vi "INI read synchronization.vi"(11 "error in (no error)":T2) -> (4 "Sync mode":T1, 6 "Trig sync en":bool, 8 "LO sync en":bool, 15 "error out":T2)   [LabVIEW 2019, in "Shared.lvlib"]
doc: "Read mmWave LOs to export"
uses:
  Shared.lvlib
  mmWave instrument_class/Sync mode.ctl
  Low-level/TypeDefs/TX trigger config.ctl
  FPGA/SubVIs/Utility/FPGA driver trigger source.ctl
  FPGA/SubVIs/Utility/FPGA driver trigger destination.ctl
  System GV.vi
  <vilib>/Utility/config.llb/NI_LVConfig.lvlib
  FPGA/SubVIs/Utility/FPGA Utility.lvlib
  mmWave instrument_class/mmWave instrument.lvclass
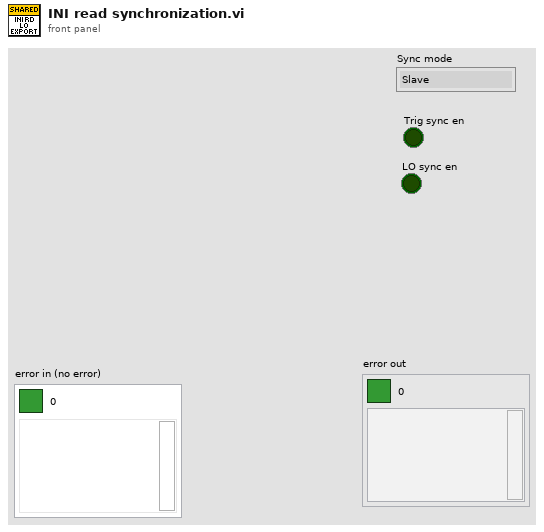
[diagram p1: front panel]
types:
  T1 = typedef "mmWave instrument.lvclass/Sync mode.ctl" = enum16{"Slave", "Master"}
  T2 = cluster{"Boolean Round":bool, "code":i32, "source":string}
  T3 = cluster{"Sync mode":T1, "Trig sync en":bool, "LO sync en":bool}
  T4 = typedef "TX trigger config.ctl" = cluster{"delay":dbl, "trig source":T5, "PXI src":i32, "export":T6, "PXI dest":i32}
  T5 = typedef "FPGA Utility.lvlib/FPGA driver trigger source.ctl" = enum16{"Use Tclk", "PXI_Trig", "Aurora RX trig"}
  T6 = typedef "FPGA Utility.lvlib/FPGA driver trigger destination.ctl" = enum16{"None", "Source trig", "Synced trig", "Delayed sync"}
  T7 = typedef "NI_LVConfig.lvlib/Config Data RefNum.ctl" = refnum<k1>
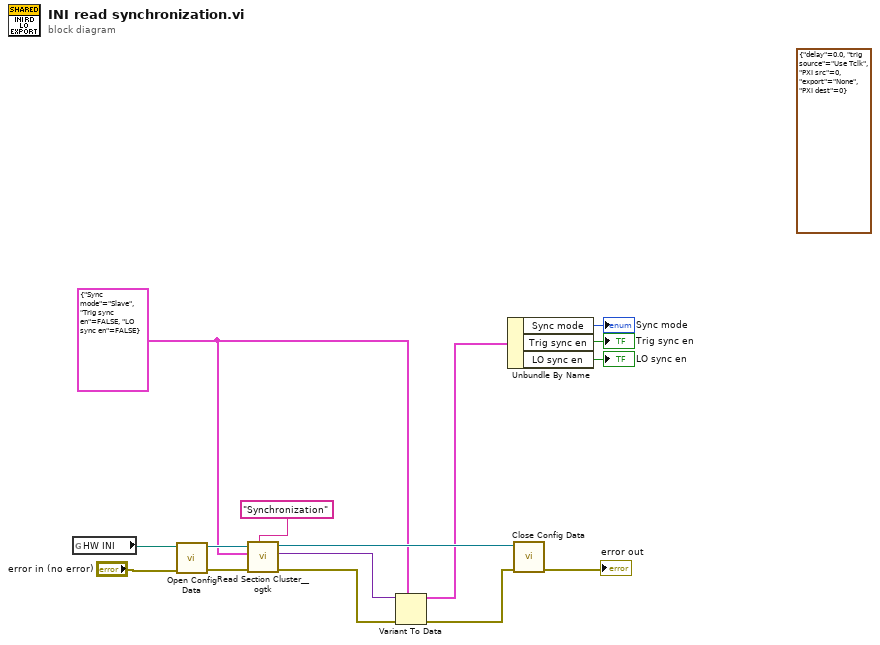
[diagram p0: block diagram]
diagram:
  w5 = T3 {"Sync mode"=enum."Slave", "Trig sync en"=FALSE, "LO sync en"=FALSE} ("LO Export")
  (unwired) T4 {"delay"=0.0, "trig source"=enum."Use Tclk", "PXI src"=0, "export"=enum."None", "PXI dest"=0} ("TX trigger options")
  n1 = global read "System GV.vi" "HW INI"() -> (w12:path)
  n2 = call <vilib>:"Open Config Data.vi"("error in (no error)"="error in (no error)", "configuration file path"=w12) -> ("error out"=w13:errorcluster, "refnum"=w15:T7)  [unwired: 7 in, 1 out]
  n3 = call <userlib>:"Read Section Cluster__ogtk.vi"("section (optional)"="Synchronization", "error in (no error)"=w13, "Section Formatted Cluster Type"=w5, "refnum"=w15) -> ("error out"=w9:errorcluster, "Section Formatted Cluster"=w10:variant, "dup refnum"=w14:T7)  [unwired: 3 in, 2 out]
  n4 = Variant To Data(error in=w9, type=w5, Variant=w10) -> (data=w4:T3, error out=w8:errorcluster)
  n5 = Unbundle By Name(w4) -> ("Sync mode"=→"Sync mode":T1, "Trig sync en"=→"Trig sync en":bool, "LO sync en"=→"LO sync en":bool)
  n6 = call <vilib>:"Close Config Data.vi"("error in (no error)"=w8, "refnum"=w14) -> ("error out"=→"error out":errorcluster)  [unwired: 8 in, 1 out]
